vi "Follower.vi"() -> ()   [LabVIEW 2016]
uses:
  <vilib>/NXT/Block Support/NXT_TimerIndex.ctl
  <vilib>/NXT/Block Support/NXT_InputPort.ctl
  <vilib>/NXT/Block Support/NXT_MessageMailbox.ctl
  <vilib>/NXT/Block Support/NXT_OutputPort.ctl
  <vilib>/NXT/Dual Mode Library/Motors/ResetMotor.vi
  <vilib>/NXT/Dual Mode Library/Sensors/EV3_Color_Reflect.vi
  <vilib>/NXT/Dual Mode Library/BT/BlueTooth_Read_num.vi
  <vilib>/NXT/NXTIO Xnodes/NXTIONodeSubVIs/NXTStopMotors.vi
  <vilib>/NXT/Dual Mode Library/Sensors/EV3_Ultrasonic_CM.vi
  <vilib>/NXT/NXTIO Xnodes/NXTIONodeSubVIs/NXTMoveMotors.vi
  <vilib>/NXT/Dual Mode Library/Display/drawText_Right.vi
  <vilib>/NXT/Dual Mode Library/Display/drawNumber.vi
  <vilib>/NXT/Dual Mode Library/Display/drawNumber_float.vi
  <vilib>/NXT/Dual Mode Library/Sensors/Touch_Pressed.vi
  <vilib>/NXT/Dual Mode Library/Sound/Tone.vi
  <vilib>/NXT/Dual Mode Library/Display/drawText.vi
  <vilib>/NXT/Subs/LVHSConnector.ctl
  <vilib>/NXT/NXTIO Xnodes/AddressXNode/NXTIOAddress.xnode
  <vilib>/NXT/NXTIO Xnodes/NXTIOXNode/NXTIO.xnode
  <vilib>/NXT/LegoClasses/BrickReference/BrickReference.lvclass
panel:
  out "Kd Chart":dbl(graph)
  out "Ki Chart":dbl(graph)
  out "Kp Chart":dbl(graph)
  out "Sensor Value Chart":sgl(graph)
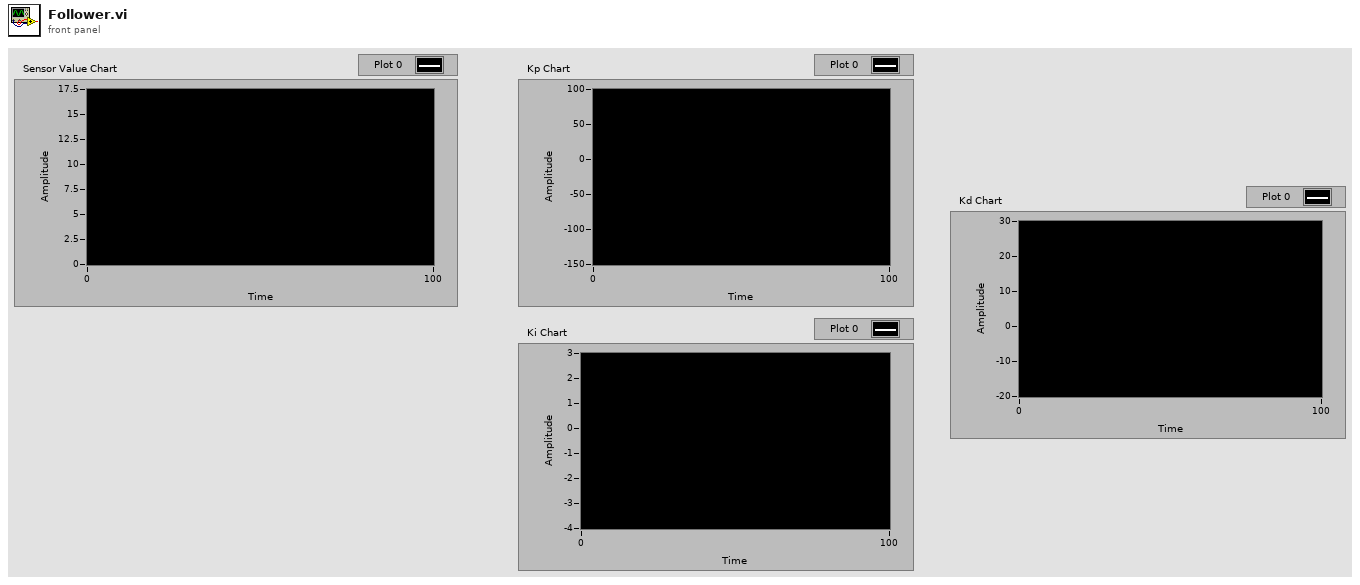
[diagram p1: front panel]
types:
  T1 = typedef "NXT_TimerIndex.ctl" = u8
  T2 = typedef "LVHSConnector.ctl" = refnum<class "BrickReference.lvclass">
  T3 = typedef "NXT_MessageMailbox.ctl" = u8
  T4 = typedef "NXT_InputPort.ctl" = u32
  T5 = typedef "NXT_OutputPort.ctl" = u8
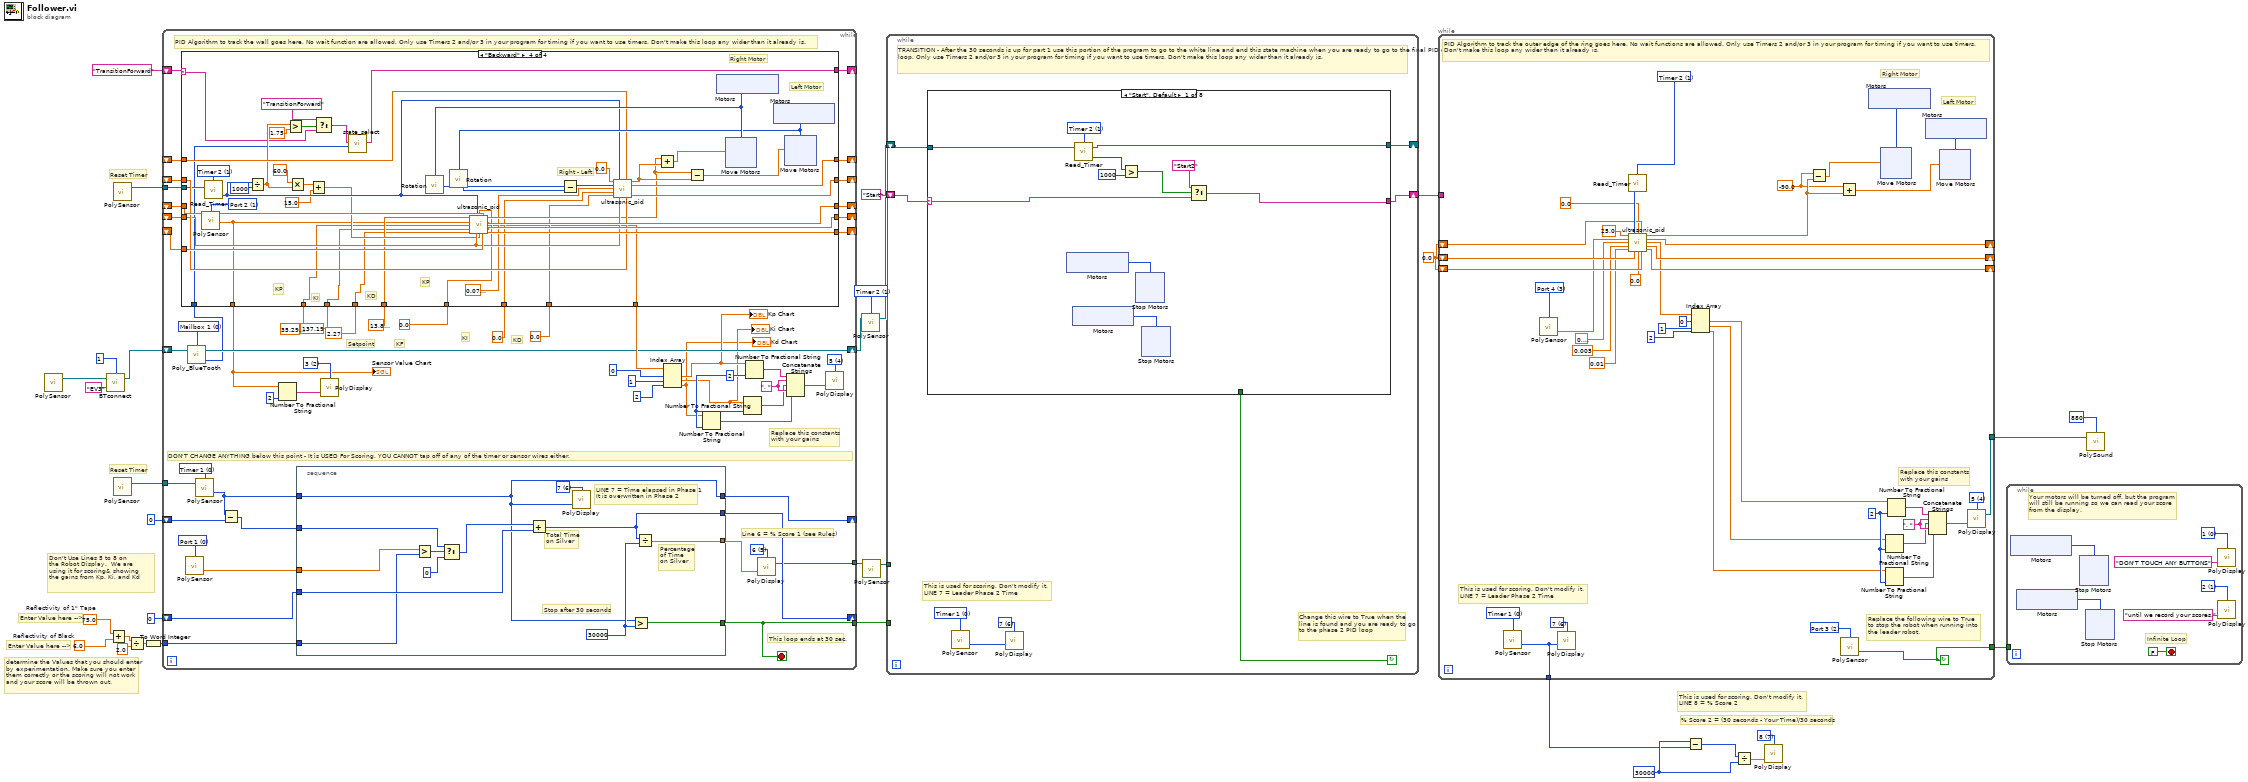
[diagram p0: block diagram]
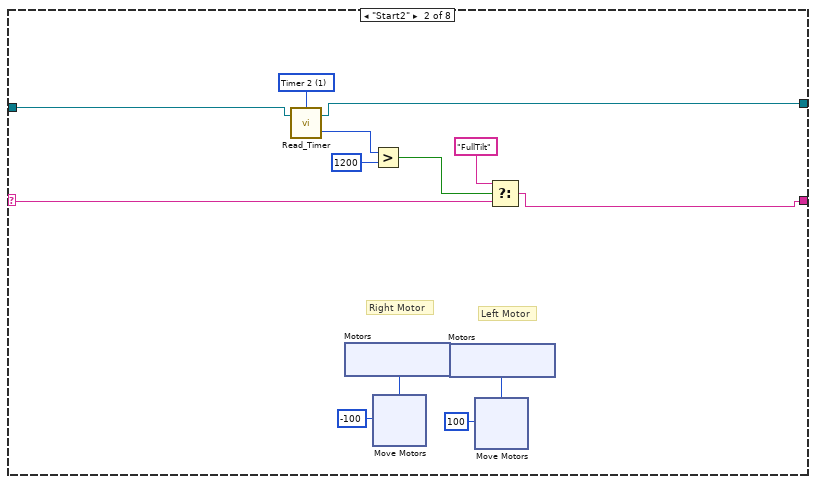
[diagram p2: hidden frame]
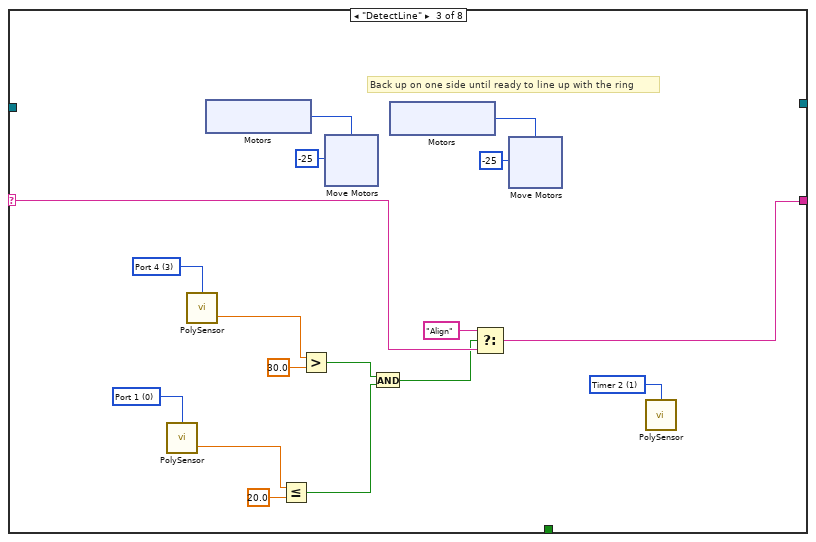
[diagram p3: hidden frame]
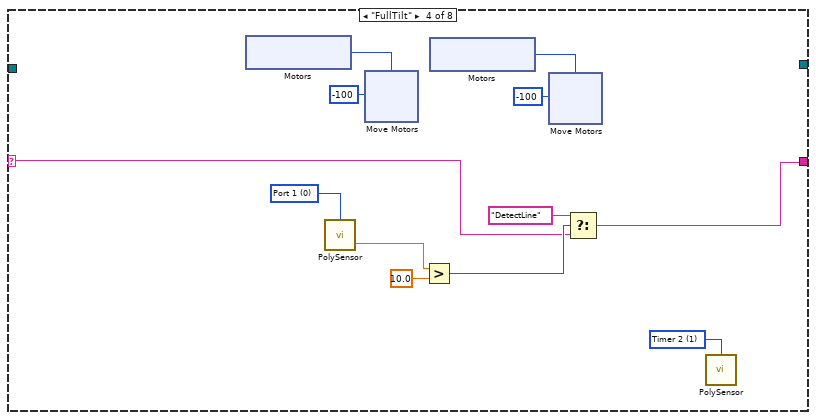
[diagram p4: hidden frame]
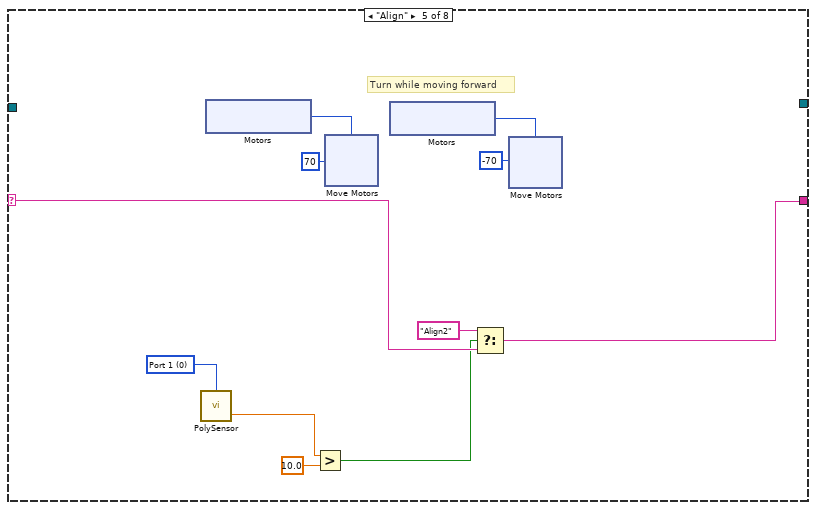
[diagram p5: hidden frame]
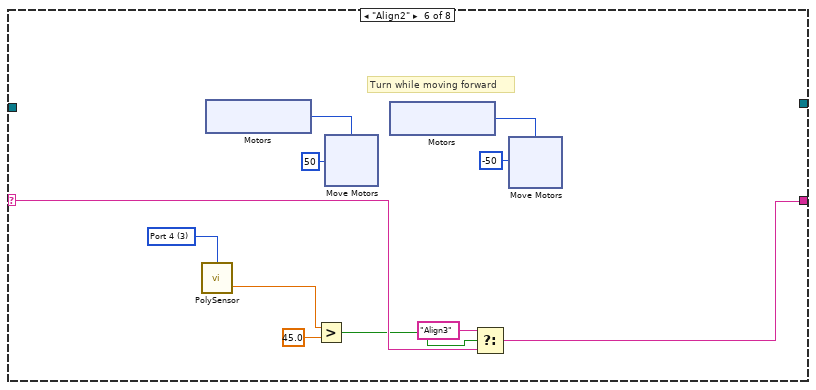
[diagram p6: hidden frame]
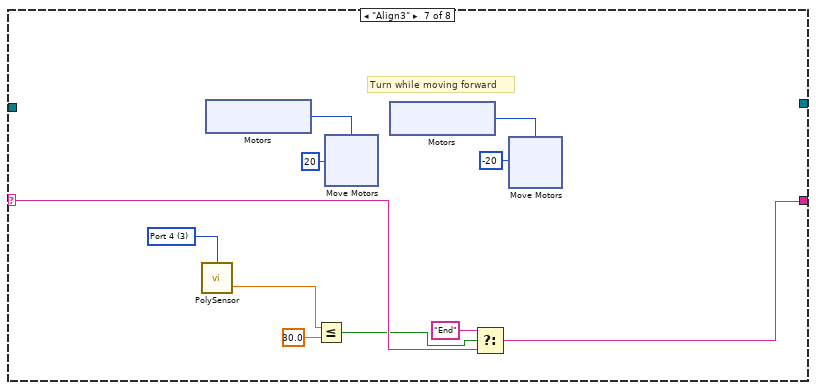
[diagram p7: hidden frame]
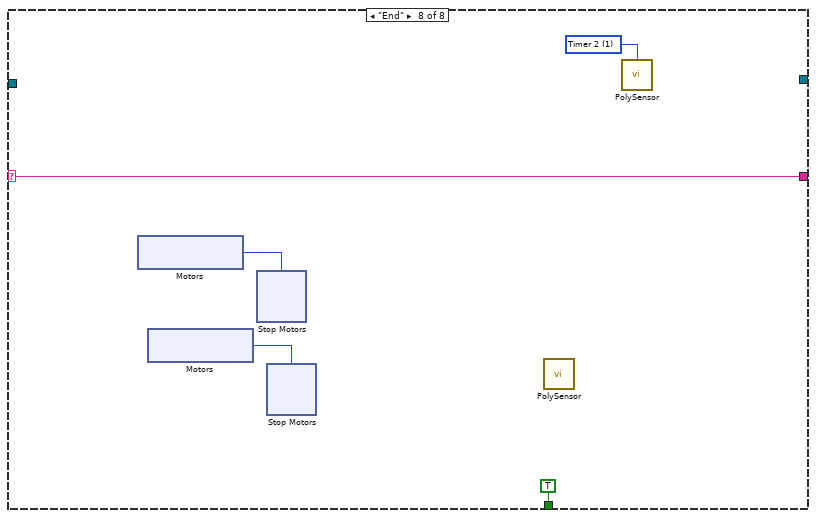
[diagram p8: hidden frame]
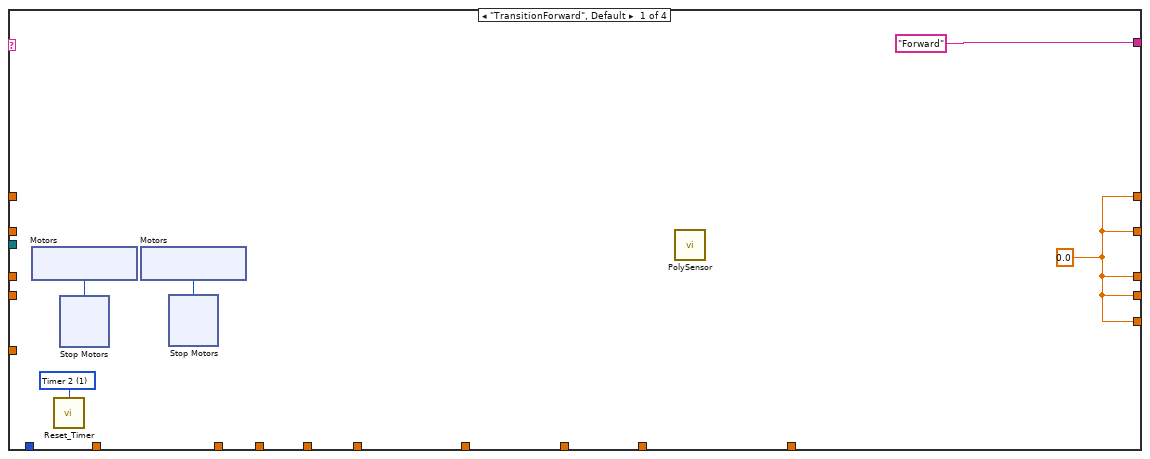
[diagram p9: hidden frame]
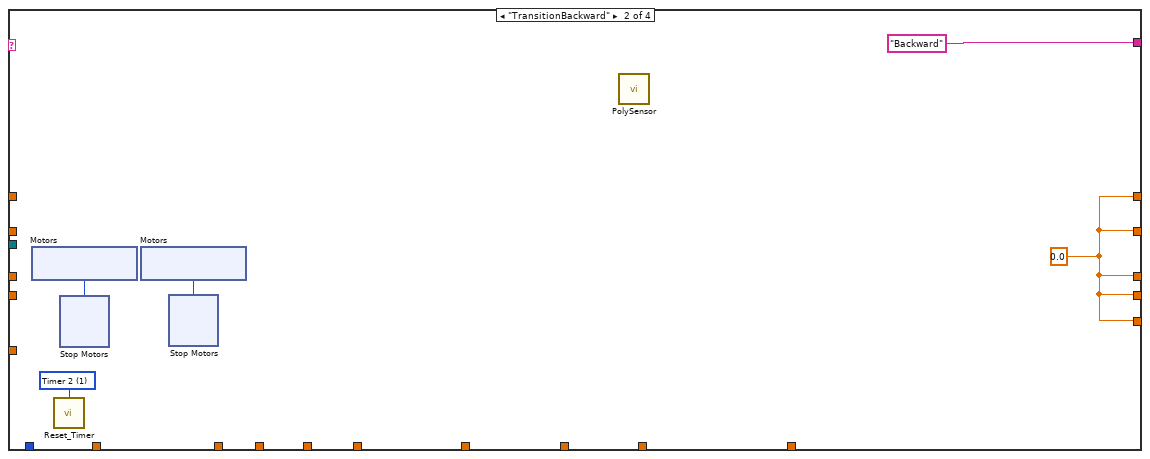
[diagram p10: hidden frame]
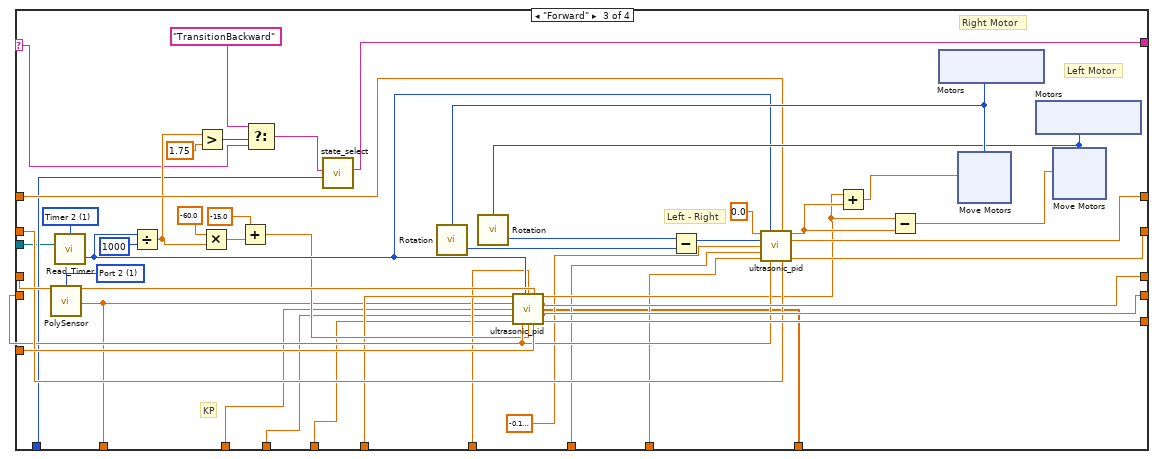
[diagram p11: hidden frame]
diagram:
  w3 = 0.0 ("Current Time")
  w10 = T1 1 items=["Timer 1", "Timer 2", "Timer 3"] ("Timer (Timer 1)")
  w16 = u32 30000 ("Value (msec)")
  w17 = i16 7 items=["1", "2", "3", "4", "5", "6", "7", "8", "9", "10", "11", "12"] ("Line")
  w23 = 6.0  # Reflectivity of Black
  w22 = 75.0  # Reflectivity of 1" Tape
  # "Reset Timer"
  # "This is used for scoring. Don't modify it.\nLINE 8 = % Score 2"
  # "Don't Use Lines 5 to 8 on\nthe Robot Display.  We are \nusing it for scoring& showing \nthe gains from Kp, Ki, and Kd"
  # "% Score 2 = (30 seconds - Your Time)/30 seconds"
  # "Enter Value here -->"
  # "determine the Values that you should enter\nby experimentation. Make sure you enter \nthem correctly or the scoring will not work\nand your score will be thrown out."
  # "Enter Value here -->"
  # "Reset Timer"
  n1 = call-poly <vilib>:"PolySensor.vi"() -> ("NXT/EV3"=w5:T2)  [unwired: 4 in]
  n2 = call <vilib>:"BTconnect.vi"("Partner Name"="EV3", "NXT/EV3"=w5, "Connection"=u8 1) -> ("NXT/EV3"=w9:T2)  [unwired: 1 out]
  n3 = Add(x=w22, y=w23) -> (x+y=w21:dbl)
  n4 = call-poly <vilib>:"PolySensor.vi"() -> ("NXT/EV3"=w4:T2)  [unwired: 4 in]
  n5 = call-poly <vilib>:"PolySensor.vi"() -> ("NXT/EV3"=w30:T2)  [unwired: 4 in]
  n6 = Divide(x=w21, y=2.0) -> (x/y=w20:dbl)
  n7 = To Word Integer(number=w20) -> (16bit integer=w27:i16)
  n8 = while {
    shift-right: [w85] -> _
    shift-left: i16 0 -> [w89]
    shift-right: [w86] -> _
    shift-left: i16 0 ("Value (msec)") -> [w88]
    tunnel: w30 -> [w84]
    tunnel: [w87] -> w29
    tunnel: w27 -> [w79]
    tunnel: [w75] -> w25
    shift-right: [w66] -> _
    shift-left: _ -> [w65]
    shift-right: [w67] -> _
    shift-left: _ -> [w64]
    shift-right: [w68] -> _
    shift-left: _ -> [w63]
    shift-right: [w62] -> _
    shift-left: _ -> [w60]
    shift-right: [w61] -> _
    shift-left: _ -> [w59]
    shift-right: [w57] -> _
    shift-left: "TransitionForward" -> [w58]
    shift-right: [w48] -> w6
    shift-left: w9 -> [w47]
    tunnel: w4 -> [w45]
    stop <- w87 stop-if-true
    w41 = i16 2 items=["1", "2", "3", "4", "5", "6", "7", "8", "9", "10", "11", "12"] ("Line")
    w46 = T3 0 items=["Mailbox 1", "Mailbox 2", "Mailbox 3", "Mailbox 4", "Mailbox 5", "Mailbox 6", "Mailbox 7", "Mailbox 8", "Mailbox 9", "Mailbox 10"] ("Mailbox")
    w71 = ", " ("string")
    w73 = i16 2 ("precision (6)")
    w74 = i16 4 items=["1", "2", "3", "4", "5", "6", "7", "8", "9", "10", "11", "12"] ("Line")
    w77 = i16 5 items=["1", "2", "3", "4", "5", "6", "7", "8", "9", "10", "11", "12"] ("Line")
    w81 = T4 0 items=["Port 1", "Port 2", "Port 3", "Port 4"] ("Port (Port 3)")
    w82 = T1 0 items=["Timer 1", "Timer 2", "Timer 3"] ("Timer (Timer 1)")
    # "KD"
    # "KI"
    # "KF"
    # "Setpoint"
    # "Replace this constants\nwith your gains"
    # "DON'T CHANGE ANYTHING below this point - It is USED For Scoring. YOU CANNOT tap off of any of the timer or sensor wires either."
    # "Line 6 = % Score 1 (see Rules)"
    # "This loop ends at 30 sec."
    # "PID Algorithm to track the wall goes here. No wait function are allowed. Only use Timers 2 and/or 3 in your program for timing if you want to use timers. Don't make this loop any wider than it already is."
    n9 = call-poly <vilib>:"PolySensor.vi"("Port (Port 1)"=w81) -> ("Scaled Value"=w80:sgl)  [unwired: 2 in, 1 out]
    n10 = call-poly <vilib>:"Poly_BlueTooth.vi"("NXT/EV3"=w47, "Mailbox"=w46) -> ("Message"=w44:i32, "NXT/EV3"=w48:T2)  [unwired: 1 in]
    n11 = case shown="\"Backward\"" w58 {
      selector: w58 -> [_ _ w132 w194]
      tunnel: [w90 w107 w169 w232] -> w68
      tunnel: [w90 w107 w168 w231] -> w67
      tunnel: [w90 w107 w167 w230] -> w66
      tunnel: w65 -> [_ _ w166 w229]
      tunnel: w64 -> [_ _ w141 w204]
      tunnel: w63 -> [_ _ w165 w228]
      tunnel: [w90 w107 w158 w221] -> w62
      tunnel: [w90 w107 w157 w220] -> w61
      tunnel: w60 -> [_ _ w155 w218]
      tunnel: w59 -> [_ _ w154 w217]
      tunnel: ["Forward" ("t") "Backward" ("t") w130 w192] -> w57
      tunnel: sgl 0.0 ("KF") -> [_ _ w137 w201]
      tunnel: sgl 13.8 ("Setpoint") -> [_ _ w138 w200]
      tunnel: 0.0 ("KI") -> [_ _ w136 w199]
      tunnel: 0.0 ("KD") -> [_ _ w135 w198]
      tunnel: [_ _ w128 w191] -> w52
      tunnel: w45 -> [_ _ w129 w196]
      tunnel: w44 -> [_ _ w133 w195]
      tunnel: [_ _ w127 w190] -> w36
      tunnel: 2.27 ("KD") -> [_ _ w126 w187]
      tunnel: 137.19 ("KI") -> [_ _ w125 w188]
      tunnel: sgl 35.29 ("KP") -> [_ _ w124 w189]
      frame "TransitionForward", Default {
        w90 = sgl 0.0 ("Error")
        w94 = T1 1 items=["Timer 1", "Timer 2", "Timer 3"] ("Timer (Timer 1)")
        n12 = xnode "Motors"() -> ("Motor"=w93:T5)
        n13 = call <vilib>:"Reset_Timer.vi"("Timer (Timer 1)"=w94) -> ()  [unwired: 3 in, 1 out]
        n14 = xnode "Stop Motors"("Motors"=w93) -> ()  [unwired: 1 in, 1 out]
        n15 = xnode "Motors"() -> ("Motor"=w92:T5)
        n16 = xnode "Stop Motors"("Motors"=w92) -> ()  [unwired: 1 in, 1 out]
        n17 = call-poly <vilib>:"PolySensor.vi"() -> ()  [unwired: 4 in, 1 out]
      }
      frame "TransitionBackward" {
        w107 = sgl 0.0 ("Error")
        w111 = T1 1 items=["Timer 1", "Timer 2", "Timer 3"] ("Timer (Timer 1)")
        n18 = xnode "Motors"() -> ("Motor"=w110:T5)
        n19 = call <vilib>:"Reset_Timer.vi"("Timer (Timer 1)"=w111) -> ()  [unwired: 3 in, 1 out]
        n20 = xnode "Stop Motors"("Motors"=w110) -> ()  [unwired: 1 in, 1 out]
        n21 = xnode "Motors"() -> ("Motor"=w109:T5)
        n22 = xnode "Stop Motors"("Motors"=w109) -> ()  [unwired: 1 in, 1 out]
        n23 = call-poly <vilib>:"PolySensor.vi"() -> ()  [unwired: 4 in, 1 out]
      }
      frame "Forward" {
        w164 = T4 1 items=["Port 1", "Port 2", "Port 3", "Port 4"] ("Port (Port 1)")
        w170 = T1 1 items=["Timer 1", "Timer 2", "Timer 3"] ("Timer (Timer 1)")
        # "Left - Right"
        # "Left Motor"
        # "Right Motor"
        # "KP"
        n24 = call-poly <vilib>:"PolySensor.vi"("Port (Port 1)"=w164) -> ("Centimeters"=w127:sgl)  [unwired: 2 in, 1 out]
        n25 = call <vilib>:"Read_Timer.vi"("NXT/EV3"=w129, "Timer (Timer 1)"=w170) -> ("Value (msec)"=w147:u32)  [unwired: 1 in, 1 out]
        n26 = Divide(x=w147, y=u32 1000) -> (x/y=w145:dbl)
        n27 = Greater?(x=w145, y=1.75) -> (0:w143:bool)
        n28 = Multiply(x=-60.0, y=w145) -> (x*y=w149:dbl)
        n29 = Add(x=-15.0, y=w149) -> (x+y=w139:dbl)
        n30 = Select(t="TransitionBackward", s=w143, f=w132) -> (s? t:f=w131:string)
        n31 = call "state_select.vi"("Mail"=w133, "Curernt State"=w131) -> ("New State"=w130:string)  [unwired: 9 in]
        n32 = call "ultrasonic_pid.vi"("Setpoint"=w138, "Time"=w147, "KF"=w137, "Error"=w165, "Input"=w127, "KP"=w124, "KI"=w125, "KD"=w126, "Previous Time"=w141, "Feed Forward"=w139, "Accumulated Error"=w166) -> ("Output"=w140:dbl, "Error"=w169:sgl, "Gains"=w128:dbl[], "Current Time"=w168:dbl, "Accumulated Error"=w167:dbl)
        n33 = xnode "Motors"() -> ("Motor"=w163:T5)
        n34 = call <vilib>:"Rotation.vi"("Port (Port A)"=w163) -> ("Angle of Rotation"=w161:i32)  [unwired: 2 in, 1 out]
        n35 = xnode "Motors"() -> ("Motor"=w162:T5)
        n36 = call <vilib>:"Rotation.vi"("Port (Port A)"=w162) -> ("Angle of Rotation"=w160:i32)  [unwired: 2 in, 1 out]
        n37 = Subtract(x=w160, y=w161) -> (x-y=w159:i32)
        n38 = call "ultrasonic_pid.vi"("Setpoint"=sgl 0.0, "Time"=w147, "Error"=w154, "Input"=w159, "KP"=sgl -0.1, "KI"=w136, "KD"=w135, "Previous Time"=w141, "Accumulated Error"=w155) -> ("Output"=w153:dbl, "Error"=w157:sgl, "Accumulated Error"=w158:dbl)  [unwired: 2 in, 2 out]
        n39 = Add(x=w140, y=w153) -> (x+y=w152:dbl)
        n40 = Subtract(x=w140, y=w153) -> (x-y=w151:dbl)
        n41 = xnode "Move Motors"("Power/Speed 1"=w152, "Motors"=w163) -> ()  [unwired: 1 in, 1 out]
        n42 = xnode "Move Motors"("Power/Speed 1"=w151, "Motors"=w162) -> ()  [unwired: 1 in, 1 out]
      }
      frame "Backward" {
        w227 = T4 1 items=["Port 1", "Port 2", "Port 3", "Port 4"] ("Port (Port 1)")
        w233 = T1 1 items=["Timer 1", "Timer 2", "Timer 3"] ("Timer (Timer 1)")
        # "KP"
        # "KD"
        # "KI"
        # "KP"
        # "Right - Left"
        # "Left Motor"
        # "Right Motor"
        n43 = call-poly <vilib>:"PolySensor.vi"("Port (Port 1)"=w227) -> ("Centimeters"=w190:sgl)  [unwired: 2 in, 1 out]
        n44 = call <vilib>:"Read_Timer.vi"("NXT/EV3"=w196, "Timer (Timer 1)"=w233) -> ("Value (msec)"=w213:u32)  [unwired: 1 in, 1 out]
        n45 = Divide(x=w213, y=u32 1000) -> (x/y=w211:dbl)
        n46 = Greater?(x=w211, y=1.75) -> (0:w209:bool)
        n47 = Multiply(x=60.0, y=w211) -> (x*y=w206:dbl)
        n48 = Add(x=w206, y=15.0 ("x")) -> (x+y=w203:dbl)
        n49 = Select(t="TransitionForward", s=w209, f=w194) -> (s? t:f=w193:string)
        n50 = call "state_select.vi"("Mail"=w195, "Curernt State"=w193) -> ("New State"=w192:string)  [unwired: 9 in]
        n51 = call "ultrasonic_pid.vi"("Setpoint"=w200, "Time"=w213, "KF"=w201, "Error"=w228, "Input"=w190, "KP"=w189, "KI"=w188, "KD"=w187, "Previous Time"=w204, "Feed Forward"=w203, "Accumulated Error"=w229) -> ("Output"=w202:dbl, "Error"=w232:sgl, "Gains"=w191:dbl[], "Current Time"=w231:dbl, "Accumulated Error"=w230:dbl)
        n52 = xnode "Motors"() -> ("Motor"=w226:T5)
        n53 = call <vilib>:"Rotation.vi"("Port (Port A)"=w226) -> ("Angle of Rotation"=w224:i32)  [unwired: 2 in, 1 out]
        n54 = xnode "Motors"() -> ("Motor"=w225:T5)
        n55 = call <vilib>:"Rotation.vi"("Port (Port A)"=w225) -> ("Angle of Rotation"=w223:i32)  [unwired: 2 in, 1 out]
        n56 = Subtract(x=w224, y=w223) -> (x-y=w222:i32)
        n57 = call "ultrasonic_pid.vi"("Setpoint"=sgl 0.0, "Time"=w213, "Error"=w217, "Input"=w222, "KP"=sgl 0.08, "KI"=w199, "KD"=w198, "Previous Time"=w204, "Accumulated Error"=w218) -> ("Output"=w216:dbl, "Error"=w220:sgl, "Accumulated Error"=w221:dbl)  [unwired: 2 in, 2 out]
        n58 = Add(x=w202, y=w216) -> (x+y=w215:dbl)
        n59 = Subtract(x=w202, y=w216) -> (x-y=w214:dbl)
        n60 = xnode "Move Motors"("Power/Speed 1"=w215, "Motors"=w226) -> ()  [unwired: 1 in, 1 out]
        n61 = xnode "Move Motors"("Power/Speed 1"=w214, "Motors"=w225) -> ()  [unwired: 1 in, 1 out]
      }
    }
    "Sensor Value Chart" <- w36
    n62 = call-poly <vilib>:"PolySensor.vi"("NXT/EV3"=w84, "Timer (Timer 1)"=w82) -> ("Value (msec)"=w83:u32)  [unwired: 1 in, 1 out]
    n63 = Subtract(x=w83, y=w88) -> (x-y=w78:u32)
    n64 = Number To Fractional String(number=w36, precision (6)=i16 2) -> (F-format string=w43:string)  [unwired: 2 in]
    n65 = stacked-sequence {
      tunnel: w89 -> [w262]
      tunnel: [w252] -> w76
      tunnel: w83 -> [w250]
      tunnel: [w261] -> w87
      tunnel: w80 -> [w256]
      tunnel: w78 -> [w258]
      tunnel: [w250] -> w86
      tunnel: [w254] -> w85
      tunnel: w79 -> [w255]
      frame #0 {
        w251 = i16 6 items=["1", "2", "3", "4", "5", "6", "7", "8", "9", "10", "11", "12"] ("Line")
        w253 = u32 30000 ("Value (msec)")
        # "LINE 7 = Time elapsed in Phase 1\nIt is overwritten in Phase 2"
        # "Percentage\nof Time\non Silver"
        # "Stop after 30 seconds"
        # "Total Time\non Silver"
        n66 = Greater?(x=w256, y=w255) -> (0:w259:bool)
        n67 = Select(t=w258, s=w259, f=i16 0) -> (s? t:f=w257:u32)
        n68 = Add(x=w257, y=w262) -> (x+y=w254:u32)
        n69 = call-poly <vilib>:"PolyDisplay.vi"("number"=w250, "Line"=w251) -> ()  [unwired: 2 in, 1 out]
        n70 = Greater?(x=w250, y=w253) -> (0:w261:bool)
        n71 = Divide(x=w254, y=w253) -> (x/y=w252:dbl)
      }
    }
    n72 = call-poly <vilib>:"PolyDisplay.vi"("Text"=w43, "Line"=w41) -> ()  [unwired: 2 in, 1 out]
    n73 = Index Array(array=w52, index #1=0 ("index"), index #2=1 ("index"), index #3=2 ("index")) -> (element #1=w39:dbl, element #2=w38:dbl, element #3=w37:dbl)
    "Kp Chart" <- w39
    "Ki Chart" <- w38
    "Kd Chart" <- w37
    n74 = Number To Fractional String(number=w37, precision (6)=w73) -> (F-format string=w69:string)  [unwired: 2 in]
    n75 = Number To Fractional String(number=w38, precision (6)=w73) -> (F-format string=w70:string)  [unwired: 2 in]
    n76 = Number To Fractional String(number=w39, precision (6)=w73) -> (F-format string=w72:string)  [unwired: 2 in]
    n77 = call-poly <vilib>:"PolyDisplay.vi"("number"=w76, "Line"=w77) -> ("NXT/EV3"=w75:T2)  [unwired: 2 in]
    n78 = Concatenate Strings(w72, w71, w70, w71, w69) -> (w40:string)
    n79 = call-poly <vilib>:"PolyDisplay.vi"("Text"=w40, "Line"=w74) -> ()  [unwired: 2 in, 1 out]
  }
  n80 = call-poly <vilib>:"PolySensor.vi"("NXT/EV3"=w6, "Timer (Timer 1)"=w10) -> ("NXT/EV3"=w11:T2)  [unwired: 2 in]
  n81 = call-poly <vilib>:"PolySensor.vi"("NXT/EV3"=w25) -> ("NXT/EV3"=w24:T2)  [unwired: 3 in]
  n82 = while {
    tunnel: w29 -> [_]
    shift-right: [w266] -> w18
    shift-left: "Start" -> [w267]
    tunnel: w24 -> [_]
    shift-right: [w263] -> _
    shift-left: w11 -> [w264]
    stop <- w265 continue-if-true
    w268 = i16 6 items=["1", "2", "3", "4", "5", "6", "7", "8", "9", "10", "11", "12"] ("Line")
    w270 = T1 0 items=["Timer 1", "Timer 2", "Timer 3"] ("Timer (Timer 1)")
    # "This is used for scoring. Don't modify it.\nLINE 7 = Leader Phase 2 Time"
    # "Change this wire to True when the line is found and you are ready to go to the phase 2 PID loop"
    # "TRANSITION - After the 30 seconds is up for part 1 use this portion of the program to go to the white line and end this state machine when you are ready to go to the final PID control loop. Only use Timers 2 and/or 3 in your program for timing if you want to use timers. Don't make this loop any wider than it already is."
    n83 = case shown="\"Start\", Default" w267 {
      selector: w267 -> [w273 w297 w335 w357 w390 w417 w444 w467]
      tunnel: [w272 w294 w333 w356 w388 w415 w442 w467] -> w266
      tunnel: [_ _ _ _ _ _ _ TRUE] -> w265
      tunnel: w264 -> [w274 w296 _ _ _ _ _ _]
      tunnel: [w271 w295 _ _ _ _ _ _] -> w263
      frame "Start", Default {
        w281 = T1 1 items=["Timer 1", "Timer 2", "Timer 3"] ("Timer (Timer 1)")
        n84 = xnode "Motors"() -> ("Motor"=w277:T5)
        n85 = xnode "Motors"() -> ("Motor"=w276:T5)
        n86 = call <vilib>:"Read_Timer.vi"("NXT/EV3"=w274, "Timer (Timer 1)"=w281) -> ("Value (msec)"=w280:u32, "NXT/EV3"=w271:T2)  [unwired: 1 in]
        n87 = Greater?(x=w280, y=u32 1000) -> (0:w279:bool)
        n88 = xnode "Stop Motors"("Motors"=w277) -> ()  [unwired: 1 in, 1 out]
        n89 = xnode "Stop Motors"("Motors"=w276) -> ()  [unwired: 1 in, 1 out]
        n90 = Select(t="Start2", s=w279, f=w273) -> (s? t:f=w272:string)
      }
      frame "Start2" {
        w306 = T1 1 items=["Timer 1", "Timer 2", "Timer 3"] ("Timer (Timer 1)")
        # "Left Motor"
        # "Right Motor"
        n91 = call <vilib>:"Read_Timer.vi"("NXT/EV3"=w296, "Timer (Timer 1)"=w306) -> ("Value (msec)"=w305:u32, "NXT/EV3"=w295:T2)  [unwired: 1 in]
        n92 = xnode "Motors"() -> ("Motor"=w301:T5)
        n93 = Greater?(x=w305, y=u32 1200) -> (0:w304:bool)
        n94 = xnode "Move Motors"("Power/Speed 1"=i8 -100, "Motors"=w301) -> ()  [unwired: 1 in, 1 out]
        n95 = xnode "Motors"() -> ("Motor"=w302:T5)
        n96 = xnode "Move Motors"("Power/Speed 1"=i8 100, "Motors"=w302) -> ()  [unwired: 1 in, 1 out]
        n97 = Select(t="FullTilt", s=w304, f=w297) -> (s? t:f=w294:string)
      }
      frame "DetectLine" {
        w324 = T4 0 items=["Port 1", "Port 2", "Port 3", "Port 4"] ("Port (Port 1)")
        w331 = T4 3 items=["Port 1", "Port 2", "Port 3", "Port 4"] ("Port (Port 1)")
        w332 = T1 1 items=["Timer 1", "Timer 2", "Timer 3"] ("Timer (Timer 1)")
        # "Back up on one side until ready to line up with the ring"
        n98 = call-poly <vilib>:"PolySensor.vi"("Port (Port 1)"=w324) -> ("Scaled Value"=w326:sgl)  [unwired: 2 in, 1 out]
        n99 = call-poly <vilib>:"PolySensor.vi"("Port (Port 1)"=w331) -> ("Scaled Value"=w329:sgl)  [unwired: 2 in, 1 out]
        n100 = xnode "Motors"() -> ("Motor"=w339:T5)
        n101 = Less Or Equal?(x=w326, y=sgl 20.0) -> (x <= y?=w323:bool)
        n102 = Greater?(x=w329, y=sgl 30.0) -> (0:w328:bool)
        n103 = xnode "Move Motors"("Power/Speed 1"=i8 -25, "Motors"=w339) -> ()  [unwired: 1 in, 1 out]
        n104 = And(x=w328, y=w323) -> (x .and. y?=w327:bool)
        n105 = xnode "Motors"() -> ("Motor"=w338:T5)
        n106 = Select(t="Align", s=w327, f=w335) -> (s? t:f=w333:string)
        n107 = xnode "Move Motors"("Power/Speed 1"=i8 -25, "Motors"=w338) -> ()  [unwired: 1 in, 1 out]
        n108 = call-poly <vilib>:"PolySensor.vi"("Timer (Timer 1)"=w332) -> ()  [unwired: 3 in, 1 out]
      }
      frame "FullTilt" {
        w358 = T1 1 items=["Timer 1", "Timer 2", "Timer 3"] ("Timer (Timer 1)")
        w359 = T4 0 items=["Port 1", "Port 2", "Port 3", "Port 4"] ("Port (Port 1)")
        n109 = xnode "Motors"() -> ("Motor"=w367:T5)
        n110 = call-poly <vilib>:"PolySensor.vi"("Port (Port 1)"=w359) -> ("Scaled Value"=w363:sgl)  [unwired: 2 in, 1 out]
        n111 = xnode "Move Motors"("Power/Speed 1"=i8 -100, "Motors"=w367) -> ()  [unwired: 1 in, 1 out]
        n112 = Greater?(x=w363, y=sgl 10.0) -> (0:w361:bool)
        n113 = xnode "Motors"() -> ("Motor"=w366:T5)
        n114 = xnode "Move Motors"("Power/Speed 1"=i8 -100, "Motors"=w366) -> ()  [unwired: 1 in, 1 out]
        n115 = Select(t="DetectLine", s=w361, f=w357) -> (s? t:f=w356:string)
        n116 = call-poly <vilib>:"PolySensor.vi"("Timer (Timer 1)"=w358) -> ()  [unwired: 3 in, 1 out]
      }
      frame "Align" {
        w387 = T4 0 items=["Port 1", "Port 2", "Port 3", "Port 4"] ("Port (Port 1)")
        # "Turn while moving forward"
        n117 = call-poly <vilib>:"PolySensor.vi"("Port (Port 1)"=w387) -> ("Scaled Value"=w385:sgl)  [unwired: 2 in, 1 out]
        n118 = xnode "Motors"() -> ("Motor"=w394:T5)
        n119 = Greater?(x=w385, y=sgl 10.0) -> (0:w384:bool)
        n120 = xnode "Move Motors"("Power/Speed 1"=i8 70, "Motors"=w394) -> ()  [unwired: 1 in, 1 out]
        n121 = xnode "Motors"() -> ("Motor"=w393:T5)
        n122 = Select(t="Align2", s=w384, f=w390) -> (s? t:f=w388:string)
        n123 = xnode "Move Motors"("Power/Speed 1"=i8 -70, "Motors"=w393) -> ()  [unwired: 1 in, 1 out]
      }
      frame "Align2" {
        w412 = T4 3 items=["Port 1", "Port 2", "Port 3", "Port 4"] ("Port (Port 1)")
        # "Turn while moving forward"
        n124 = call-poly <vilib>:"PolySensor.vi"("Port (Port 1)"=w412) -> ("Scaled Value"=w414:sgl)  [unwired: 2 in, 1 out]
        n125 = xnode "Motors"() -> ("Motor"=w421:T5)
        n126 = Greater?(x=w414, y=sgl 45.0) -> (0:w411:bool)
        n127 = xnode "Move Motors"("Power/Speed 1"=i8 50, "Motors"=w421) -> ()  [unwired: 1 in, 1 out]
        n128 = xnode "Motors"() -> ("Motor"=w420:T5)
        n129 = Select(t="Align3", s=w411, f=w417) -> (s? t:f=w415:string)
        n130 = xnode "Move Motors"("Power/Speed 1"=i8 -50, "Motors"=w420) -> ()  [unwired: 1 in, 1 out]
      }
      frame "Align3" {
        w439 = T4 3 items=["Port 1", "Port 2", "Port 3", "Port 4"] ("Port (Port 1)")
        # "Turn while moving forward"
        n131 = call-poly <vilib>:"PolySensor.vi"("Port (Port 1)"=w439) -> ("Scaled Value"=w441:sgl)  [unwired: 2 in, 1 out]
        n132 = xnode "Motors"() -> ("Motor"=w448:T5)
        n133 = Less Or Equal?(x=w441, y=sgl 30.0) -> (x <= y?=w438:bool)
        n134 = xnode "Move Motors"("Power/Speed 1"=i8 20, "Motors"=w448) -> ()  [unwired: 1 in, 1 out]
        n135 = xnode "Motors"() -> ("Motor"=w447:T5)
        n136 = Select(t="End", s=w438, f=w444) -> (s? t:f=w442:string)
        n137 = xnode "Move Motors"("Power/Speed 1"=i8 -20, "Motors"=w447) -> ()  [unwired: 1 in, 1 out]
      }
      frame "End" {
        w468 = T1 1 items=["Timer 1", "Timer 2", "Timer 3"] ("Timer (Timer 1)")
        n138 = xnode "Motors"() -> ("Motor"=w466:T5)
        n139 = xnode "Motors"() -> ("Motor"=w465:T5)
        n140 = xnode "Stop Motors"("Motors"=w466) -> ()  [unwired: 1 in, 1 out]
        n141 = xnode "Stop Motors"("Motors"=w465) -> ()  [unwired: 1 in, 1 out]
        n142 = call-poly <vilib>:"PolySensor.vi"() -> ()  [unwired: 4 in, 1 out]
        n143 = call-poly <vilib>:"PolySensor.vi"("Timer (Timer 1)"=w468) -> ()  [unwired: 3 in, 1 out]
      }
    }
    n144 = call-poly <vilib>:"PolySensor.vi"("Timer (Timer 1)"=w270) -> ("Value (msec)"=w269:u32)  [unwired: 2 in, 1 out]
    n145 = call-poly <vilib>:"PolyDisplay.vi"("number"=w269, "Line"=w268) -> ()  [unwired: 2 in, 1 out]
  }
  n146 = while {
    tunnel: [w484] -> w19
    tunnel: w18 -> [_]
    tunnel: [w521] -> w15
    shift-right: [w506] -> _
    shift-left: w3 -> [w500]
    shift-right: [w507] -> _
    shift-left: w3 -> [w501]
    shift-right: [w508] -> _
    shift-left: w3 -> [w503]
    tunnel: [w482] -> w2
    stop <- w484 continue-if-true
    w485 = -90.0 ("y")
    w494 = T4 2 items=["Port 1", "Port 2", "Port 3", "Port 4"] ("Port (Port 1)")
    w499 = T4 3 items=["Port 1", "Port 2", "Port 3", "Port 4"] ("Port (Port 1)")
    w505 = T1 1 items=["Timer 1", "Timer 2", "Timer 3"] ("Timer (Timer 1)")
    w517 = ", " ("string")
    w519 = i16 2 ("precision (6)")
    w520 = i16 4 items=["1", "2", "3", "4", "5", "6", "7", "8", "9", "10", "11", "12"] ("Line")
    w522 = i16 6 items=["1", "2", "3", "4", "5", "6", "7", "8", "9", "10", "11", "12"] ("Line")
    w523 = T1 0 items=["Timer 1", "Timer 2", "Timer 3"] ("Timer (Timer 1)")
    # "Left Motor"
    # "Right Motor"
    # "Replace this constants\nwith your gains"
    # "This is used for scoring. Don't modify it.\nLINE 7 = Leader Phase 2 Time"
    # "PID Algorithm to track the outer edge of the ring goes here. No wait functions are allowed. Only use Timers 2 and/or 3 in your program for timing if you want to use timers.\nDon't make this loop any wider than it already is."
    # "Replace the following wire to True\nto stop the robot when running into \nthe leader robot."
    n147 = call-poly <vilib>:"PolySensor.vi"("Timer (Timer 1)"=w523) -> ("Value (msec)"=w521:u32)  [unwired: 2 in, 1 out]
    n148 = call-poly <vilib>:"PolySensor.vi"("Port (Port 1)"=w499) -> ("Scaled Value"=w498:sgl)  [unwired: 2 in, 1 out]
    n149 = call-poly <vilib>:"PolyDisplay.vi"("number"=w521, "Line"=w522) -> ()  [unwired: 2 in, 1 out]
    n150 = call <vilib>:"Read_Timer.vi"("Timer (Timer 1)"=w505) -> ("Value (msec)"=w504:u32)  [unwired: 2 in, 1 out]
    n151 = call "ultrasonic_pid.vi"("Setpoint"=sgl 25.0, "Time"=w504, "KF"=sgl 0.0, "Error"=w500, "Input"=w498, "KP"=sgl 0.7, "KI"=0.005, "KD"=0.01, "Previous Time"=w501, "Feed Forward"=sgl 0.0, "Accumulated Error"=w503) -> ("Output"=w486:dbl, "Error"=w506:sgl, "Gains"=w493:dbl[], "Current Time"=w507:dbl, "Accumulated Error"=w508:dbl)
    n152 = Index Array(array=w493, index #1=0 ("index"), index #2=1 ("index"), index #3=2 ("index")) -> (element #1=w489:dbl, element #2=w488:dbl, element #3=w487:dbl)
    n153 = Subtract(x=w485, y=w486) -> (x-y=w511:dbl)
    n154 = Add(x=w485, y=w486) -> (x+y=w510:dbl)
    n155 = call-poly <vilib>:"PolySensor.vi"("Port (Port 1)"=w494) -> ("Yes / No"=w484:bool)  [unwired: 2 in, 1 out]
    n156 = xnode "Motors"() -> ("Motor"=w513:T5)
    n157 = xnode "Move Motors"("Power/Speed 1"=w511, "Motors"=w513) -> ()  [unwired: 1 in, 1 out]
    n158 = Number To Fractional String(number=w488, precision (6)=w519) -> (F-format string=w516:string)  [unwired: 2 in]
    n159 = Number To Fractional String(number=w487, precision (6)=w519) -> (F-format string=w515:string)  [unwired: 2 in]
    n160 = Number To Fractional String(number=w489, precision (6)=w519) -> (F-format string=w518:string)  [unwired: 2 in]
    n161 = xnode "Motors"() -> ("Motor"=w512:T5)
    n162 = Concatenate Strings(w518, w517, w516, w517, w515) -> (w514:string)
    n163 = xnode "Move Motors"("Power/Speed 1"=w510, "Motors"=w512) -> ()  [unwired: 1 in, 1 out]
    n164 = call-poly <vilib>:"PolyDisplay.vi"("Text"=w514, "Line"=w520) -> ("NXT/EV3"=w482:T2)  [unwired: 2 in]
  }
  n165 = Subtract(x=w16, y=w15) -> (x-y=w14:u32)
  n166 = Divide(x=w14, y=w16) -> (x/y=w13:dbl)
  n167 = call-poly <vilib>:"PolyDisplay.vi"("number"=w13, "Line"=w17) -> ()  [unwired: 2 in, 1 out]
  n168 = while {
    tunnel: w19 -> [_]
    stop <- FALSE stop-if-true
    w540 = i16 1 items=["1", "2", "3", "4", "5", "6", "7", "8", "9", "10", "11", "12"] ("Line")
    w543 = i16 0 items=["1", "2", "3", "4", "5", "6", "7", "8", "9", "10", "11", "12"] ("Line")
    # "Your motors will be turned off, but the program\nwill still be running so we can read your score\nfrom the display."
    # "Infinite Loop"
    n169 = xnode "Motors"() -> ("Motor"=w545:T5)
    n170 = xnode "Motors"() -> ("Motor"=w544:T5)
    n171 = xnode "Stop Motors"("Motors"=w545) -> ()  [unwired: 1 in, 1 out]
    n172 = xnode "Stop Motors"("Motors"=w544) -> ()  [unwired: 1 in, 1 out]
    n173 = call-poly <vilib>:"PolyDisplay.vi"("Text"="DON'T TOUCH ANY BUTTONS", "Line"=w543) -> ()  [unwired: 2 in, 1 out]
    n174 = call-poly <vilib>:"PolyDisplay.vi"("Text"="until we record your scores.", "Line"=w540) -> ()  [unwired: 2 in, 1 out]
  }
  n175 = call-poly <vilib>:"PolySound.vi"("NXT/EV3"=w2, "Tone (440 Hz)"=u16 880) -> ()  [unwired: 2 in, 1 out]
